vi "Unregister Subsystem.vi"(8 "error in (no error)":errorcluster, 9 "RegistryKey":string, 10 "JKI SMO":refnum<class "SMO.lvclass">) -> (0 "error out":errorcluster, 2 "JKI SMO out":refnum<class "SMO.lvclass">)   [LabVIEW 2019, in "Registry-SMO.lvclass"]
doc: "JKI State Machine Objects (SMO) 1.3.0.56\nJKI - JKI\nCopyright (c) 2017, JKI"
uses:
  Registry-SMO.lvclass
  SMO/SMO.lvclass
  Registry-SMO.lvclass/Registry-SMO.ctl
  Support/Attribute.Identity/Attribute.Identity.lvclass/Attribute.Identity.ctl
  Support/Attribute.Identity/Attribute.Identity.lvclass
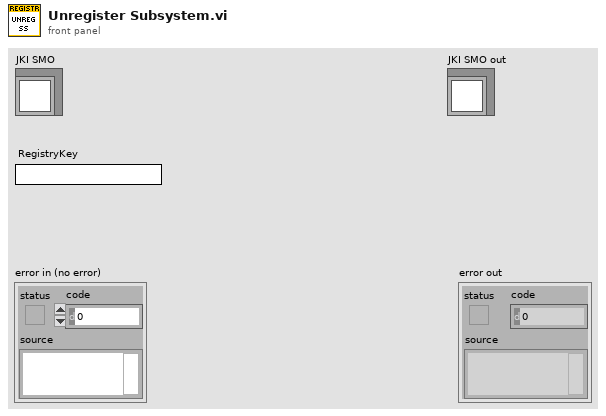
[diagram p1: front panel]
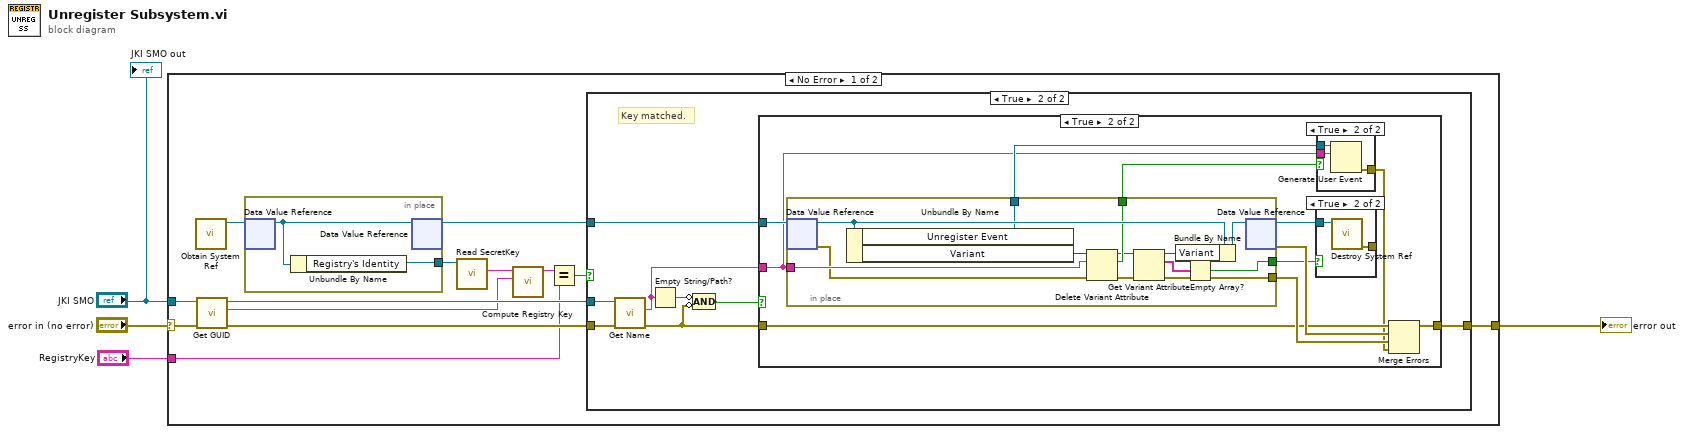
[diagram p0: block diagram]
diagram:
  n1 = case shown="No Error" "error in (no error)" {
    selector: "error in (no error)" -> [w16 w59]
    tunnel: [w17 w59] -> w3
    tunnel: "JKI SMO" -> [w14 _]
    tunnel: "RegistryKey" -> [w6 _]
    frame No Error {
      n2 = call "Obtain System Ref.vi"() -> ("JKI SMO System"=w12:refnum<data-value>)  [unwired: 10 in, 1 out]
      n3 = call "Get GUID.vi"("error in (no error)"=w16, "SMO"=w14) -> ("error out"=w15:errorcluster, "GUID"=w8:string, "SMO out"=w13:refnum<class "SMO.lvclass">)  [unwired: 7 in]
      n4 = in-place {
        in-place-border: [w57] -> w10
        n5 = in-place-dvr #1(w12) -> (w58:refnum<class "Registry-SMO.lvclass">)  [unwired: 1 out]
        n6 = Unbundle By Name(w58) -> ("Registry's Identity"=w57:refnum<class "Attribute.Identity.lvclass">)
        n7 = in-place-dvr #1(w58) -> (w11:refnum<data-value>)  [unwired: 1 out]
      }
      n8 = call "Read SecretKey.vi"("Attribute.Identity in"=w10) -> ("SecretKey"=w9:string)  [unwired: 8 in, 2 out]
      n9 = call "Compute Registry Key.vi"("SMO GUID"=w8, "Registry's SecretKey"=w9) -> ("Registry Key"=w7:string)  [unwired: 9 in]
      n10 = Equal?(x=w7, y=w6) -> (x = y?=w5:bool)
      n11 = case shown="True" w5 {
        tunnel: [w18 w26] -> w17
        tunnel: w15 -> [w18 w21]
        tunnel: w13 -> [_ w20]
        tunnel: w11 -> [_ w19]
        frame False {
          # "Registry Key does not match. Cannot unregister SMO"
        }
        frame True {
          # "Key matched."
          n12 = call "Get Name.vi"("error in (no error)"=w21, "SMO"=w20) -> ("error out"=w22:errorcluster, "Name"=w25:string)  [unwired: 7 in, 1 out]
          n13 = Empty String/Path?(string/path=w25) -> (empty?=w24:bool)
          n14 = Compound Arithmetic op=AND(invert w24, invert w22) -> (w23:bool)
          n15 = case shown="True" w23 {
            tunnel: [w27 w36] -> w26
            tunnel: w25 -> [_ w31]
            tunnel: w22 -> [w27 w34]
            tunnel: w19 -> [_ w35]
            frame False {
            }
            frame True {
              n16 = in-place {
                in-place-border: w31 -> [w53]
                in-place-border: [w46] -> w37
                in-place-border: [w51] -> w32
                in-place-border: [w50] -> w30
                in-place-border: [w44] -> w28
                n17 = in-place-dvr #2(w35) -> (w56:refnum<class "Registry-SMO.lvclass">, w52:errorcluster)
                n18 = Unbundle By Name(w56) -> ("Unregister Event"=w51:refnum<user-event>, "Variant"=w54:variant)
                n19 = Delete Variant Attribute(4:w52, 6:w53, 7:w54) -> (0:w47:errorcluster, 2:w50:bool, 3:w49:variant)
                n20 = Get Variant Attribute(Variant=w49, error in=w47) -> (duplicate Variant=w48:variant, names=w45:string[], error out=w46:errorcluster)  [unwired: 2 in, 1 out]
                n21 = Bundle By Name(cluster=w56, "Variant"=w48) -> (w55:refnum<class "Registry-SMO.lvclass">)
                n22 = Empty Array?(array=w45) -> (empty?=w44:bool)
                n23 = in-place-dvr #2(w55) -> (w29:refnum<data-value>, w38:errorcluster)
              }
              n24 = case shown="True" w28 {
                tunnel: w29 -> [_ w40]
                tunnel: [_ w39] -> _
                frame False {
                }
                frame True {
                  n25 = call "Destroy System Ref.vi"("JKI SMO System"=w40) -> ("error out"=w39:errorcluster)  [unwired: 10 in]
                }
              }
              n26 = case shown="True" w30 {
                tunnel: [_ w43] -> w33
                tunnel: w32 -> [_ w42]
                tunnel: w31 -> [_ w41]
                frame False {
                }
                frame True {
                  n27 = Generate User Event(user event=w42, event data cluster=w41) -> (error out=w43:errorcluster)  [unwired: 2 in, 1 out]
                }
              }
              n28 = Merge Errors(w34, w38, w37, w33) -> (w36:errorcluster)
            }
          }
        }
      }
    }
    frame Error {
    }
  }
  "error out" <- w3
  "JKI SMO out" <- "JKI SMO"
